vi "AcquireData.vi"(8 "error in (no error)":errorcluster, 11 "MCSA acquisition config":T5 {"FixedSizeX31"."InputConfig" items=["AC Coupled", "DC Coupled", "IEPE AC Coupled"]}) -> (0 "error out":errorcluster, 1 "dataflow messages":T1[](array[typedef]), 3 "MCSA acquisition config out":T5 {"FixedSizeX31"."InputConfig" items=["AC Coupled", "DC Coupled", "IEPE AC Coupled"]})   [LabVIEW 2017, in "McsaFpgaAcquisition.lvlib"]
uses:
  <vilib>/addons/InsightCM/Devices/Shared/Mcsa/McsaFpgaAcquisition/McsaFpgaAcquisition.lvlib
  <vilib>/addons/InsightCM/Devices/Shared/Mcsa/McsaFpgaAcquisition/controls/Configuration.ctl
  <vilib>/addons/InsightCM/Devices/Shared/Cms/CmsAcquisition/controls/FixedSizeArrays.ctl
  <vilib>/LabVIEW Targets/FPGA/cRIO/shared/nicrio_ModuleControls/nicrio_cRIO-9232_ConfigModeRing.ctl
  <vilib>/addons/InsightCM/Devices/Shared/Cms/cRIOWfmAcq/subVIs/RIO Wfm Cust Ctrls/rwfm_SamplingInfo.ctl
  <vilib>/addons/InsightCM/Devices/Shared/Mcsa/McsaFpgaAcquisition/controls/Group.ctl
  <vilib>/addons/InsightCM/Devices/Shared/Mcsa/McsaFpgaAcquisition/controls/ChannelMcsa.ctl
  <vilib>/addons/InsightCM/Devices/Shared/Mcsa/McsaFpgaAcquisition/controls/RangeParams.ctl
  <vilib>/addons/InsightCM/Devices/Shared/Common/DataFlow/controls/Data.ctl
  <vilib>/addons/InsightCM/Utilities/DataAccessors/controls/wfmSGL_DVR.ctl
  <vilib>/addons/PointValueMap/controls/PointMap.ctl
  <vilib>/addons/InsightCM/Devices/Shared/Common/DataFlow/controls/Type.ctl
  <vilib>/addons/PointValueMap/PointValueMap.lvlib
  <vilib>/addons/InsightCM/Devices/Shared/Common/DataFlow/DataFlow.lvlib
  <vilib>/addons/InsightCM/Devices/Shared/Cms/cRIOWfmAcq/cRIOWfmLib.lvlib
  <vilib>/addons/InsightCM/Devices/Shared/Cms/CmsAcquisition/CmsAcquisition.lvlib
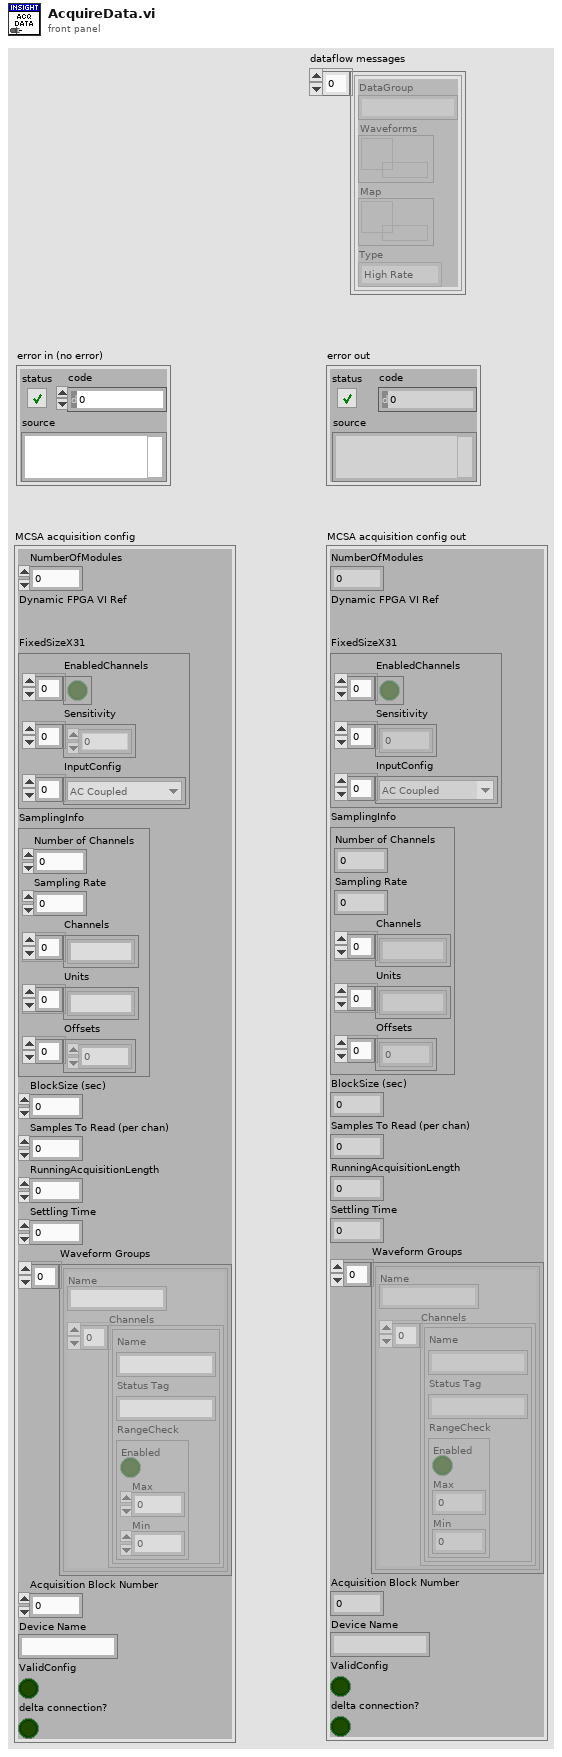
[diagram p1: front panel]
types:
  T1 = typedef "DataFlow.lvlib/Data.ctl" = cluster{"DataGroup":string, "Waveforms":T2, "Map":T3, "Type":T4}
  T2 = typedef "wfmSGL_DVR.ctl" = refnum<data-value>
  T3 = typedef "PointValueMap.lvlib/PointMap.ctl" = refnum<data-value>
  T4 = typedef "DataFlow.lvlib/Type.ctl" = enum16{"High Rate", "Low Rate", "Burst Mode"}
  T5 = typedef "McsaFpgaAcquisition.lvlib/Configuration.ctl" = cluster{"NumberOfModules":i16, "Dynamic FPGA VI Ref":refnum<k20>, "FixedSizeX31":T6, "SamplingInfo":T8, "BlockSize (sec)":dbl, "Samples To Read (per chan)":i32, "RunningAcquisitionLength":dbl, "Settling Time":dbl, "Waveform Groups":T9[], "Acquisition Block Number":i32, "Device Name":string, "ValidConfig":bool, "delta connection?":bool}
  T6 = typedef "CmsAcquisition.lvlib/FixedSizeArrays.ctl" = cluster{"EnabledChannels":bool[], "Sensitivity":dbl[], "InputConfig":T7[]}
  T7 = typedef "nicrio_cRIO-9232_ConfigModeRing.ctl" = u8
  T8 = typedef "cRIOWfmLib.lvlib/rwfm_SamplingInfo.ctl" = cluster{"Number of Channels":i32, "Sampling Rate":dbl, "Channels":string[], "Units":string[], "Offsets":sgl[]}
  T9 = typedef "McsaFpgaAcquisition.lvlib/Group.ctl" = cluster{"Name":string, "Channels":T10[]}
  T10 = typedef "McsaFpgaAcquisition.lvlib/ChannelMcsa.ctl" = cluster{"Name":string, "Status Tag":string, "RangeCheck":T11}
  T11 = typedef "McsaFpgaAcquisition.lvlib/RangeParams.ctl" = cluster{"Enabled":bool, "Max":dbl, "Min":dbl}
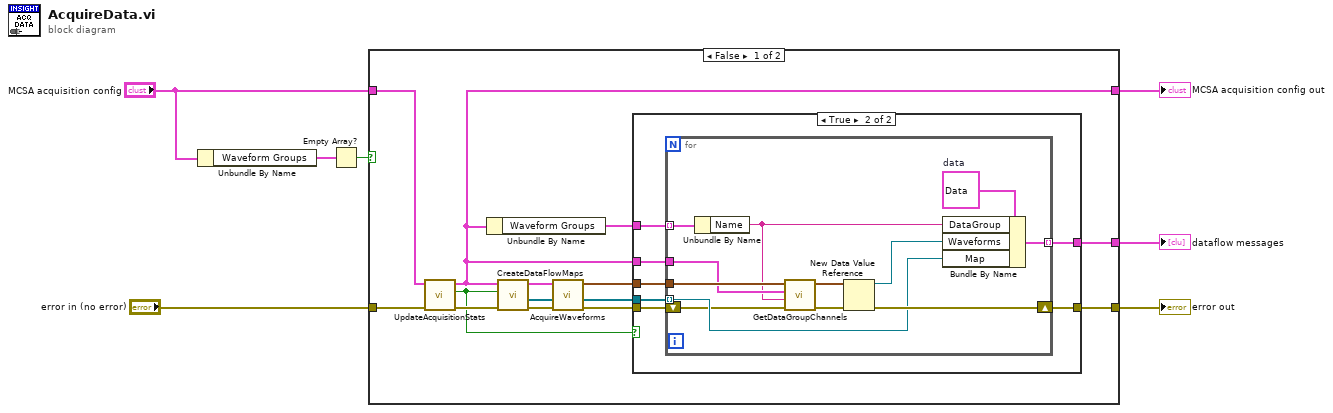
[diagram p0: block diagram]
diagram:
  n1 = Unbundle By Name("MCSA acquisition config") -> ("Waveform Groups"=w3:T9[])
  n2 = Empty Array?(array=w3) -> (empty?=w1:bool)
  n3 = case shown="False" w1 {
    tunnel: "MCSA acquisition config" -> [w20 w43]
    tunnel: [w8 w43] -> w7
    tunnel: [w13 w42] -> w6
    tunnel: [w12 _] -> w5
    tunnel: "error in (no error)" -> [w11 w42]
    frame False {
      n4 = call <vilib>:"UpdateAcquisitionStats.vi"("error in (no error)"=w11, "configuration"=w20) -> ("error out"=w19:errorcluster, "settling time requirement met?"=w9:bool, "configuration"=w8:T5)  [unwired: 7 in]
      n5 = Unbundle By Name(w8) -> ("Waveform Groups"=w21:T9[])
      n6 = call <vilib>:"CreateDataFlowMaps.vi"("error in (no error)"=w19, "settling time met"=w9, "MCSA Acquisition Config"=w8) -> ("error out"=w15:errorcluster, "maps"=w17:T3[], "MCSA Acquisition Config out"=w18:T5)  [unwired: 6 in]
      n7 = call <vilib>:"AcquireWaveforms.vi"("error in (no error)"=w15, "Data Flow Maps"=w17, "MCSA Acquisition Config"=w18) -> ("error out"=w14:errorcluster, "Data Flow Maps out"=w16:T3[], "Waveforms"=w10:waveform(sgl)[])  [unwired: 6 in]
      n8 = case shown="True" w9 {
        tunnel: w21 -> [_ w29]
        tunnel: w16 -> [_ w28]
        tunnel: w14 -> [w22 w27]
        tunnel: [w22 w26] -> w13
        tunnel: [_ w25] -> w12
        tunnel: w10 -> [_ w24]
        tunnel: w8 -> [_ w23]
        frame False {
        }
        frame True {
          n9 = for {
            tunnel: w29 -> [w41] mode=indexing
            tunnel: w24 -> [w35]
            tunnel: w28 -> [w37] mode=indexing
            tunnel: [w40] -> w25 mode=indexing
            shift-right: [w38] -> w26
            shift-left: w27 -> [w34]
            tunnel: w23 -> [w31]
            w39 = T1 {"DataGroup"="", "Waveforms"=refnum, "Map"=refnum, "Type"=enum."High Rate"}  # data
            n10 = Unbundle By Name(w41) -> ("Name"=w30:string)
            n11 = call <vilib>:"GetDataGroupChannels.vi"("error in (no error)"=w34, "group"=w30, "923x acquisition config"=w31, "all waveforms"=w35) -> ("error out"=w33:errorcluster, "this groups channels"=w32:waveform(sgl)[])  [unwired: 6 in]
            n12 = New Data Value Reference(data value=w32, error in=w33) -> (data value reference=w36:refnum<data-value>, error out=w38:errorcluster)
            n13 = Bundle By Name(cluster=w39, "DataGroup"=w30, "Waveforms"=w36, "Map"=w37) -> (w40:T1)
          }
        }
      }
    }
    frame True {
    }
  }
  "error out" <- w6
  "MCSA acquisition config out" <- w7
  "dataflow messages" <- w5
